vi "encodeBooleanRaw.vi"(3 "Boolean":bool) -> (1 "MessagePackRaw":u8)   [LabVIEW 2015, in "MsgPack.lvlib"]
uses:
  MsgPack.lvlib
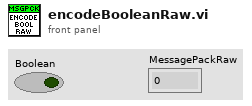
[diagram p1: front panel]
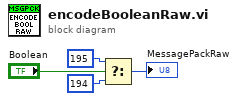
[diagram p0: block diagram]
diagram:
  n1 = Select(t=u8 195, s="Boolean", f=u8 194) -> (s? t:f=→"MessagePackRaw":u8)
